vi "SpecAn Common Configure.vi"(0 "RFmx Handle In":refnum<k21>, 1 "Selector String":string, 5 "RFmx SpecAn Spectrum Configuration":T1={"Center Frequency (Hz)"=1000000000.0, "Reference Level (dBm)"=0.0, "External Attenuation (dB)"=0.0, "Digital Edge Source"="PXI_Trig0", "Digital Edge"=0, "Trigger Delay (s)"=0.0, "Enable Trigger?"=TRUE, "Frequency Reference Source"="PXI_Clk", "SelectedPorts"="", "Auto Level Enabled"=FALSE, "Auto Level Measurement Interval (s)"=0.01, "Auto Level Bandwidth (Hz)"=20000000.0} {"Auto Level Bandwidth (Hz)" format="%#_6p"; "Auto Level Measurement Interval (s)" format="%#_6p"; "Trigger Delay (s)" format="%.2p"; "Digital Edge" items=["Rising Edge", "Falling Edge"]; "External Attenuation (dB)" format="%.2f"; "Reference Level (dBm)" format="%.2f"; "Center Frequency (Hz)" format="%.6p"}, 11 "error in (no error)":errorcluster) -> (4 "RFmx Handle Out":refnum<k21>, 15 "error out":errorcluster)   [LabVIEW 2016, in "RFmxSpecAn.lvlib"]
uses:
  RFmxSpecAn.lvlib
  Typedefs/SpecAn Common Configuration.ctl
  <vilib>/RFmx/SpecAn/mx/RFmxSpecAn.llb/RFmxSpecAn Configure Digital Edge Trigger.vi
  <resource>/objmgr/RFmxSpecAn.rc
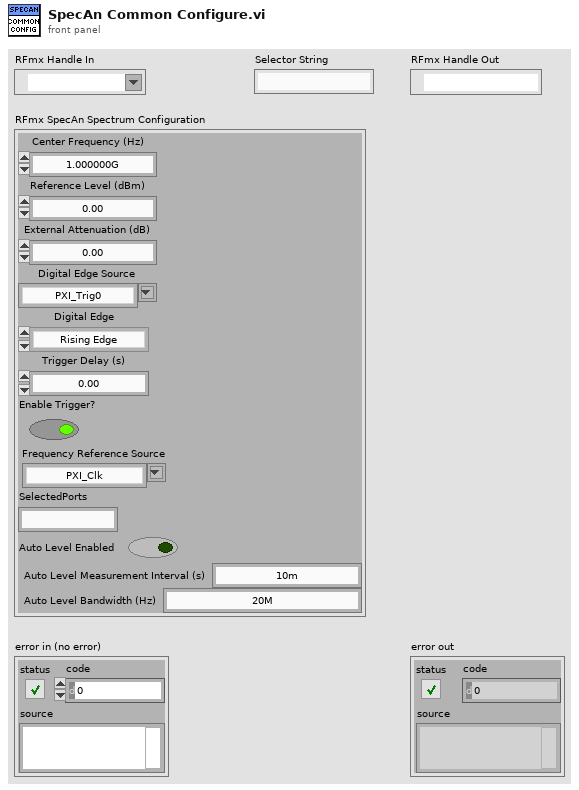
[diagram p1: front panel]
types:
  T1 = typedef "RFmxSpecAn.lvlib/SpecAn Common Configuration.ctl" = cluster{"Center Frequency (Hz)":dbl, "Reference Level (dBm)":dbl, "External Attenuation (dB)":dbl, "Digital Edge Source":string, "Digital Edge":i32, "Trigger Delay (s)":dbl, "Enable Trigger?":bool, "Frequency Reference Source":string, "SelectedPorts":string, "Auto Level Enabled":bool, "Auto Level Measurement Interval (s)":dbl, "Auto Level Bandwidth (Hz)":dbl}
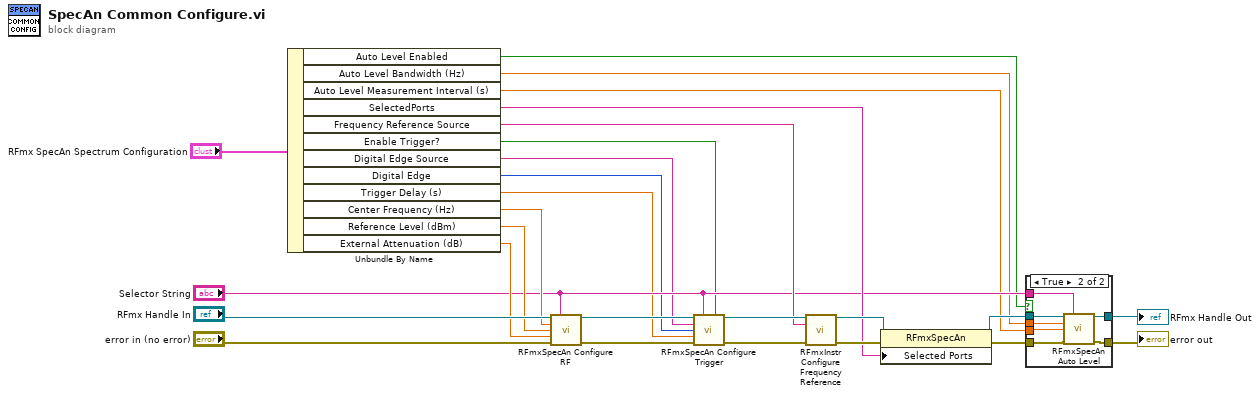
[diagram p0: block diagram]
diagram:
  n1 = Unbundle By Name("RFmx SpecAn Spectrum Configuration") -> ("Auto Level Enabled"=w7:bool, "Auto Level Bandwidth (Hz)"=w6:dbl, "Auto Level Measurement Interval (s)"=w5:dbl, "SelectedPorts"=w13:string, "Frequency Reference Source"=w15:string, "Enable Trigger?"=w4:bool, "Digital Edge Source"=w3:string, "Digital Edge"=w2:i32, "Trigger Delay (s)"=w1:dbl, "Center Frequency (Hz)"=w22:dbl, "Reference Level (dBm)"=w21:dbl, "External Attenuation (dB)"=w20:dbl)
  n2 = call <vilib>:"RFmxSpecAn Configure RF.vi"("Instrument Handle In"="RFmx Handle In", "Selector String"="Selector String", "Center Frequency (Hz)"=w22, "Reference Level"=w21, "External Attenuation (dB)"=w20, "error in (no error)"="error in (no error)") -> ("Instrument Handle Out"=w26:refnum<k21>, "error out"=w25:errorcluster)  [unwired: 8 in]
  n3 = call-poly <vilib>:"RFmxSpecAn Configure Trigger.vi"("Instrument Handle In"=w26, "Selector String"="Selector String", "Enable Trigger?"=w4, "Digital Edge Source"=w3, "Digital Edge"=w2, "Trigger Delay (s)"=w1, "error in (no error)"=w25) -> ("Instrument Handle Out"=w17:refnum<k21>, "error out"=w18:errorcluster)  [unwired: 7 in]
  n4 = call <vilib>:"RFmxInstr Configure Frequency Reference.vi"("Instrument Handle In"=w17, "Frequency Reference Source"=w15, "error in (no error)"=w18) -> ("Instrument Handle Out"=w16:refnum<k21>, "error out"=w14:errorcluster)  [unwired: 11 in]
  n5 = property class="RFmxSpecAn"(reference=w16, error in=w14, "Selected Ports"=w13) -> (reference out=w12:refnum<k21>, error out=w10:errorcluster)
  n6 = case shown="True" w7 {
    tunnel: w12 -> [w28 w35]
    tunnel: [w28 w34] -> w11
    tunnel: w10 -> [w27 w33]
    tunnel: [w27 w32] -> w9
    tunnel: "Selector String" -> [_ w31]
    tunnel: w6 -> [_ w30]
    tunnel: w5 -> [_ w29]
    frame False {
    }
    frame True {
      n7 = call <vilib>:"RFmxSpecAn Auto Level.vi"("Instrument Handle In"=w35, "Selector String"=w31, "Bandwidth (Hz)"=w30, "Measurement Interval (s)"=w29, "error in (no error)"=w33) -> ("Instrument Handle Out"=w34:refnum<k21>, "error out"=w32:errorcluster)  [unwired: 8 in, 1 out]
    }
  }
  "error out" <- w9
  "RFmx Handle Out" <- w11
